vi "OP500Z8_VG_progressBar_P.vi"() -> ()   [LabVIEW 2020]
panel:
  out "progression":u8(slide) scale=0.0..100.0
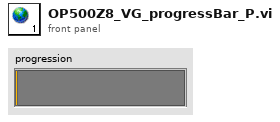
[diagram p1: front panel]
diagram:
